vi "Get XYZ Voltage.vi"(8 "error in (no error)":errorcluster, 11 "hdl in":i32) -> (0 "error out":errorcluster, 1 "Get Y voltage(V)":dbl, 2 "Get X voltage(V)":dbl, 3 "hdl":i32, 4 "Get Z voltage(V)":dbl)   [LabVIEW 2011, in "Thorlabs_MDT69xB.lvlib"]
doc: "Get xyz voltage, only valid for MDT693B three channel controller."
uses:
  <instrlib>/Thorlabs_MDT69xB/Thorlabs_MDT69xB.lvlib
  <instrlib>/Thorlabs_MDT69xB/Data/MDT_COMMAND_LIB_win32.dll
  <instrlib>/Thorlabs_MDT69xB/Data/MDT_COMMAND_LIB_x64.dll
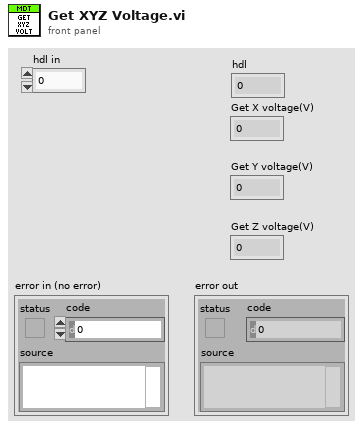
[diagram p1: front panel]
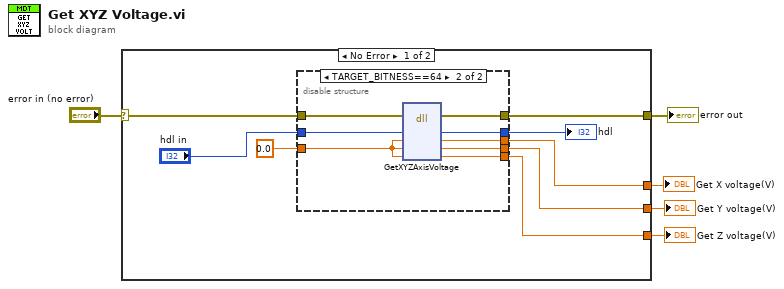
[diagram p0: block diagram]
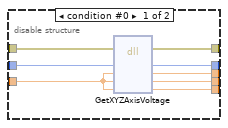
[diagram p2: hidden frame]
diagram:
  n1 = case shown="No Error" "error in (no error)" {
    selector: "error in (no error)" -> [w13 w30]
    tunnel: [w10 w30] -> w4
    tunnel: [w11 _] -> w3
    tunnel: [w7 _] -> w2
    tunnel: [w6 _] -> w1
    frame No Error {
      n2 = disable-structure shown="TARGET_BITNESS==64" {
        disable-tunnel: w13 -> [w21 w29]
        disable-tunnel: "hdl in" -> [w20 w28]
        disable-tunnel: [w19 w27] -> w11
        disable-tunnel: [w18 w26] -> w10
        disable-tunnel: [w17 w25] -> w9
        disable-tunnel: 0.0 ("voltage") -> [w16 w24]
        disable-tunnel: [w15 w23] -> w7
        disable-tunnel: [w14 w22] -> w6
        frame condition #0 {
          n3 = dll-call lib="E:/Program Files (x86)/National Instruments/LabVIEW 2011/instr.lib/Thorlabs_MDT69xB/Data/MDT_COMMAND_LIB_win32.dll" fn="GetXYZAxisVoltage"(error in=w21, "hdl"=w20, "X voltage"=w16, "Y voltage"=w16, "Z voltage"=w16) -> (error out=w18:errorcluster, "hdl"=w17:i32, "X voltage"=w19:dbl, "Y voltage"=w14:dbl, "Z voltage"=w15:dbl)  [unwired: 3 in, 1 out]
        }
        frame condition #1 (active) {
          n4 = dll-call lib="C:/Program Files/National Instruments/LabVIEW 2011/instr.lib/Thorlabs_MDT69xB/Data/MDT_COMMAND_LIB_x64.dll" fn="GetXYZAxisVoltage"(error in=w29, "hdl"=w28, "X voltage"=w24, "Y voltage"=w24, "Z voltage"=w24) -> (error out=w26:errorcluster, "hdl"=w25:i32, "X voltage"=w27:dbl, "Y voltage"=w22:dbl, "Z voltage"=w23:dbl)  [unwired: 3 in, 1 out]
        }
      }
      "hdl" <- w9
    }
    frame Error {
    }
  }
  "error out" <- w4
  "Get X voltage(V)" <- w3
  "Get Y voltage(V)" <- w1
  "Get Z voltage(V)" <- w2
